vi "Construct Sequence.vi"(8 "error in":errorcluster, 11 "cPAS Sequence Builder in":refnum<class "cPAS Sequence Builder.lvclass">) -> (0 "error out":errorcluster, 2 "New Sequence":refnum<class "SEQ.lvclass">, 3 "cPAS Sequence Builder out":refnum<class "cPAS Sequence Builder.lvclass">)   [LabVIEW 2012, in "cPAS Sequence Builder.lvclass"]
doc: "Construct a new sequence using the builder class."
uses:
  cPAS Sequence Builder.lvclass
  Reusable/Sequence/STEPS/LEAVES/Double/Switch DBL.lvclass
  Reusable/Sequence/SEQ/SEQ.lvclass
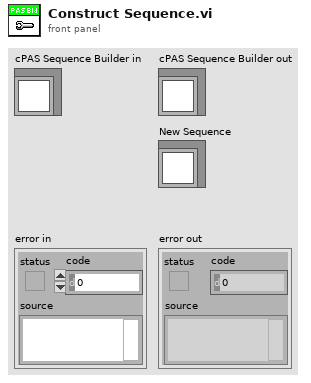
[diagram p1: front panel]
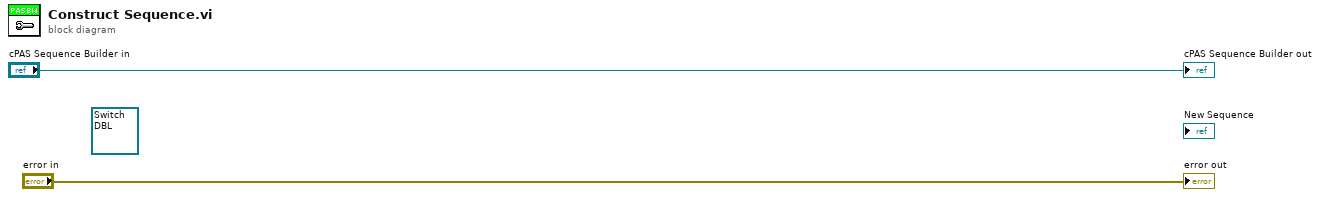
[diagram p0: block diagram]
diagram:
  (unwired) refnum<class "Switch DBL.lvclass"> refnum ("Sequence Composition:Switch DBL")
  "error out" <- "error in"
  "cPAS Sequence Builder out" <- "cPAS Sequence Builder in"
